vi "PrimaryAttackerRole_init.vi"(8 "error in (no error)":errorcluster, 11 "PrimaryAttackerRole in":refnum<class "PrimaryAttackerRole.lvclass">) -> (0 "error out":errorcluster, 3 "PrimaryAttackerRole out":refnum<class "PrimaryAttackerRole.lvclass">)   [LabVIEW 2023, in "PrimaryAttackerRole.lvclass"]
uses:
  PrimaryAttackerRole.lvclass
  C:/Users/ebert/Documents/codes/SSL/repo/SSL_AI/NewSTP/NewRoles/Role_v2_class/Role_v2.lvclass
  PrimaryAttackerRole.lvclass/PrimaryAttackerRole.ctl
  NewSTP/NewRoles/Role_v2_class/Role_v2.lvclass
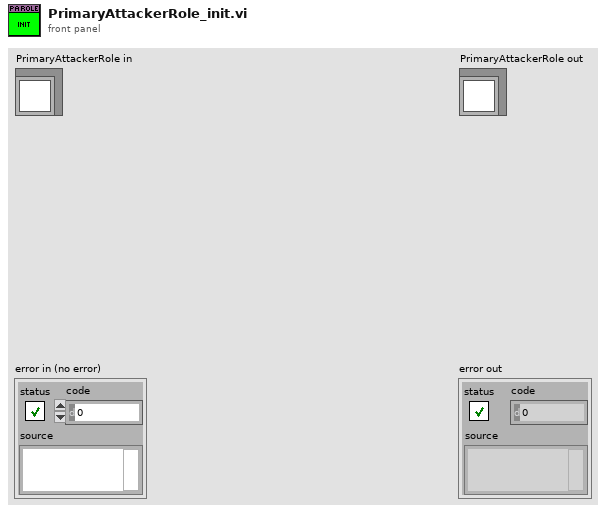
[diagram p1: front panel]
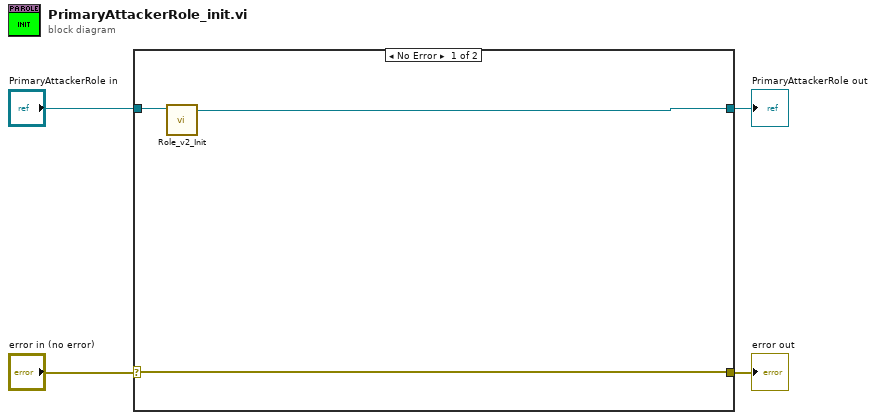
[diagram p0: block diagram]
diagram:
  n1 = case shown="No Error" "error in (no error)" {
    selector: "error in (no error)" -> [w7 w9]
    tunnel: [w7 w9] -> w3
    tunnel: [w5 w8] -> w1
    tunnel: "PrimaryAttackerRole in" -> [w6 w8]
    frame No Error {
      n2 = call "Role_v2_Init.vi"("object in"=w6) -> ("object out"=w5:refnum<class "PrimaryAttackerRole.lvclass">)  [unwired: 17 in, 1 out]
    }
    frame Error {
    }
  }
  "error out" <- w3
  "PrimaryAttackerRole out" <- w1
